vi "SPI read many.vi"(8 "error in (no error)":errorcluster, 9 "Addresses":u8[](array[numeric]), 10 "spi configuration in":T2, 11 "Device ref in":T1) -> (0 "error out":errorcluster, 1 "read data":u8[](array[numeric]), 2 "spi configuration out":T2, 3 "Device ref out":T1)   [LabVIEW 2013]
uses:
  <vilib>/ni845x/ni845x.llb/ni845xSpiConfiguration.ctl
  <vilib>/ni845x/ni845x.llb/ni845xControl.ctl
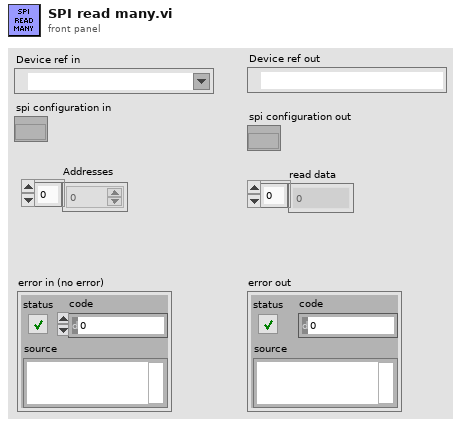
[diagram p1: front panel]
types:
  T1 = typedef "ni845xControl.ctl" = refnum<k21>
  T2 = typedef "ni845xSpiConfiguration.ctl" = refnum<k20>
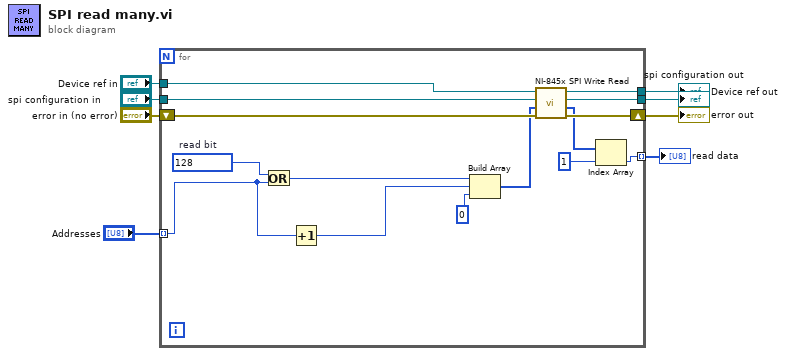
[diagram p0: block diagram]
diagram:
  n1 = for {
    tunnel: [w22] -> w2
    tunnel: [w21] -> w3
    tunnel: "spi configuration in" -> [w19]
    tunnel: "Device ref in" -> [w18]
    tunnel: [w11] -> w5 mode=indexing
    tunnel: "Addresses" -> [w10] mode=indexing
    shift-right: [w23] -> w1
    shift-left: "error in (no error)" -> [w20]
    w17 = u8 128  # read bit
    n2 = Or(x=w17, y=w10) -> (x .or. y?=w16:u8)
    n3 = Increment(x=w10) -> (x+1=w9:u8)
    n4 = Build Array(w16, w9, u8 0 ("element")) -> (w14:u8[])
    n5 = call <vilib>:"NI-845x SPI Write Read.vi"("error in (no error)"=w20, "write data"=w14, "spi configuration in"=w19, "device reference in"=w18) -> ("error out"=w23:errorcluster, "read data"=w13:u8[], "spi configuration out"=w22:T2, "device reference out"=w21:T1)  [unwired: 4 in]
    n6 = Index Array(array=w13, index=1) -> (element=w11:u8)
  }
  "error out" <- w1
  "spi configuration out" <- w2
  "Device ref out" <- w3
  "read data" <- w5
